vi "Vision Processing.vi"(4 "error in (no error)":errorcluster) -> ()   [LabVIEW 2011]
doc: "This VI runs in parallel to other tasks. It gets images from the camera, processes them for color or shape and use that information to affect robot behavior."
uses:
  <vilib>/vision/NI_Vision_Development_Module.lvlib
  VisionData.vi
  <vilib>/Rock Robotics/WPI/Camera/WPI_CameraImageSize.ctl
panel:
  in  "Color Mode":u16(ring)=1 items=["RGB", "HSL", "HSV", "HSI"]
  in  "Blue/Lum":cluster{"Lower value":i32, "Upper value":i32}={"Lower value"=40, "Upper value"=255}
  in  "Green/Sat":cluster{"Lower value":i32, "Upper value":i32}={"Lower value"=100, "Upper value"=255}
  in  "Red/hue":cluster{"Lower value":i32, "Upper value":i32}={"Lower value"=237, "Upper value"=8}
  in  "milliseconds to wait":u32=10
  out "x-y":u32
  in  "Compression":i32 min=0 max=100
  in  "Image Size":T1=enum."320x240"
  out "VisionClusterOut":T2
  out "Boolean":bool
  out "IRLLeft":bool
  out "IRLCenter":bool
  out "IRLRight":bool
  out "output array":bool[](array[boolean])
  out "error out":errorcluster
  in  "ActuallyDrawRectangles":bool
  in  "Enable/Disable Vision":bool=TRUE
  out "Scored Particle Info 3":T3(array[cluster])
  out "Scored Particle Info 2":T3(array[cluster])
  out "Scored Particle Info":T3(array[cluster])
  out "Processed Image 2":T4(plugin-control)
  in  "Score Limits":T5={"Rect Coverage"=60.0, "Aspect Ratio"=40.0, "X Edge Strength"=40.0, "Y Edge Strength"=60.0}
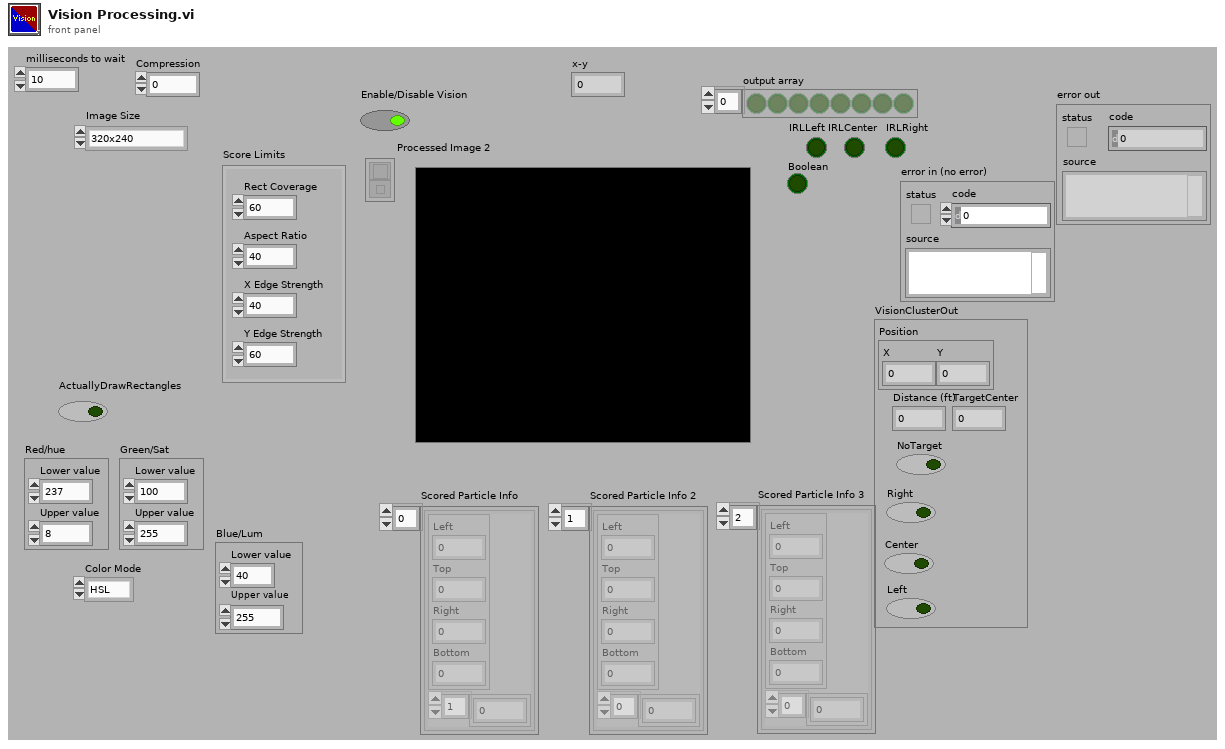
[diagram p1: front panel]
types:
  T1 = typedef "WPI_CameraImageSize.ctl" = enum16{"640x480", "320x240", "160x120"}
  T2 = cluster{"Position":cluster{"X":dbl, "Y":dbl}, "Distance (ft)":dbl, "NoTarget":bool, "Right":bool, "Center":bool, "Left":bool, "TargetCenter":dbl}
  T3 = cluster{cluster{"Left":dbl, "Top":dbl, "Right":dbl, "Bottom":dbl}, dbl[]}[]
  T4 = typedef "IMAQ Image.ctl" = refnum<image>
  T5 = cluster{"Rect Coverage":dbl, "Aspect Ratio":dbl, "X Edge Strength":dbl, "Y Edge Strength":dbl}
  T6 = typedef "Image Type" = u32
  T7 = typedef "WPI_CameraDevRef.ctl" = cluster{"Camera Address":string, "CameraStatus":errorcluster, "Acquire Image Notifier":refnum<notifier>}
  T8 = typedef "WPI_DigitalOutputDevRef.ctl" = cluster{"Digital Module":T9, "DIO Channel":T10, "DevStatus":errorcluster}
  T9 = typedef "FPGA_TypedefDigitalModule.ctl" = enum16{"Digital Module 1", "Digital Module 2"}
  T10 = typedef "FPGA_DIOChannel.ctl" = enum8{"DIO 1", "DIO 2", "DIO 3", "DIO 4", "DIO 5", "DIO 6", "DIO 7", "DIO 8", "DIO 9", "DIO 10", "DIO 11", "DIO 12", "DIO 13", "DIO 14", "Invalid"}
  T11 = cluster{"Position":cluster{"X":dbl, "Y":dbl}, "Distance (ft)":dbl, "NoTarget":bool, "Right":bool, "Center":bool, "Left":bool, "TargetCenter":dbl}[]
  T12 = cluster{"Avg. Horizontal ":dbl, "Avg Vertical":dbl}[]
  T13 = cluster{"Left":dbl, "Top":dbl, "Right":dbl, "Bottom":dbl}
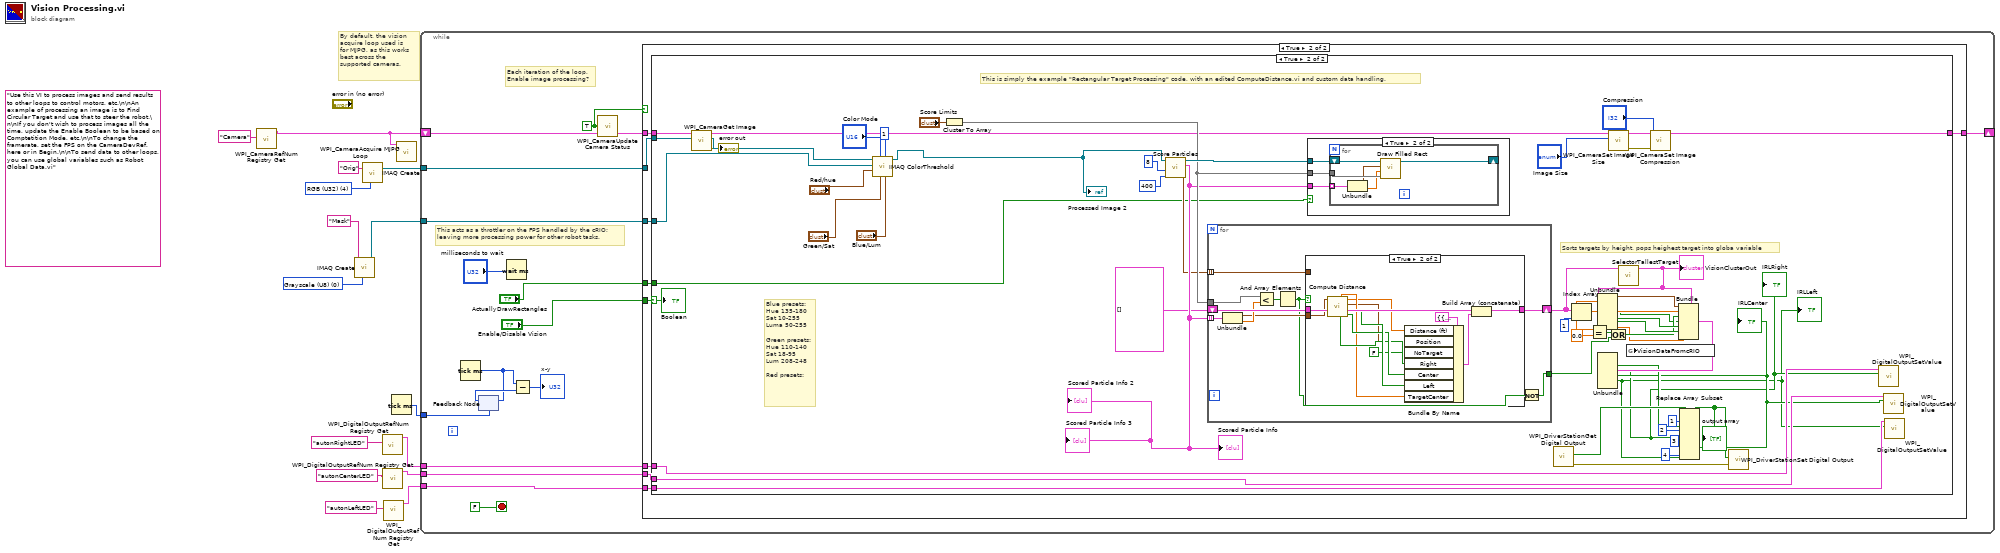
[diagram p0: block diagram]
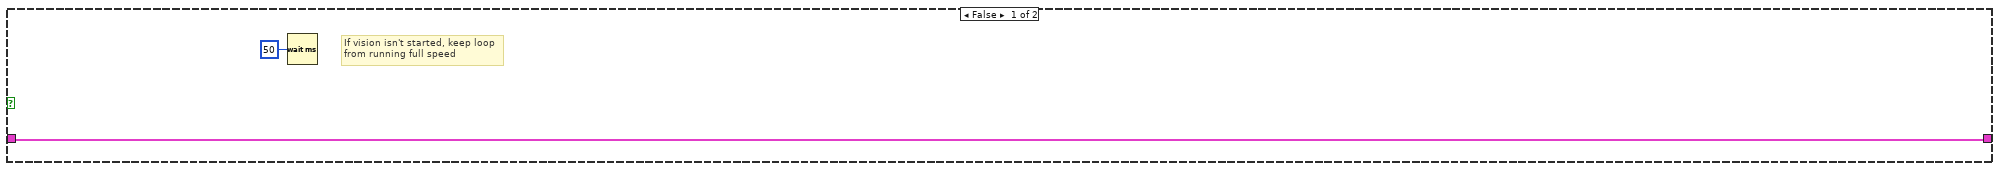
[diagram p2: hidden frame]
diagram:
  w11 = T6 0 items=["Grayscale (U8)", "Grayscale (I16)", "Grayscale (SGL)", "Complex (CSG)", "RGB (U32)", "HSL (U32)", "RGB (U64)"] ("Image Type")
  (unwired) "Use this VI to process images and send results to other loops to control motors, etc.\n\nAn example of processing an image is to Find Circular Target and use that to steer the robot.\n\nIf you don't wish to process images all the time, update the Enable Boolean to be based on Comptetition Mode, etc.\n\nTo change the framerate, set the FPS on the CameraDevRef, here or in Begin.\n\nTo send data to other loops, you can use global variables such as Robot Global Data.vi"
  w15 = T6 4 items=["Grayscale (U8)", "Grayscale (I16)", "Grayscale (SGL)", "Complex (CSG)", "RGB (U32)", "HSL (U32)", "RGB (U64)"] ("Image Type")
  # "By default, the vision\nacquire loop used is\nfor MJPG, as this works\nbest across the\nsupported cameras."
  n1 = call <vilib>:"WPI_CameraRefNum Registry Get.vi"("refnum name"="Camera") -> ("CameraDevRef"=w9:T7)  [unwired: 9 in, 1 out]
  n2 = call "IMAQ Create"("Image Name"="Mask", "Image Type"=w11) -> ("New Image"=w10:T4)  [unwired: 2 in, 2 out]
  n3 = call "IMAQ Create"("Image Name"="Orig", "Image Type"=w15) -> ("New Image"=w13:T4)  [unwired: 2 in, 2 out]
  n4 = call <vilib>:"WPI_DigitalOutputRefNum Registry Get.vi"("refnum name"="autonRightLED") -> ("DigitalOutputDevRef"=w4:T8)  [unwired: 9 in, 1 out]
  n5 = call <vilib>:"WPI_DigitalOutputRefNum Registry Get.vi"("refnum name"="autonCenterLED") -> ("DigitalOutputDevRef"=w3:T8)  [unwired: 9 in, 1 out]
  n6 = call <vilib>:"WPI_DigitalOutputRefNum Registry Get.vi"("refnum name"="autonLeftLED") -> ("DigitalOutputDevRef"=w2:T8)  [unwired: 9 in, 1 out]
  n7 = Tick Count (ms)() -> (millisecond timer value=w1:u32)
  n8 = call <vilib>:"WPI_CameraAcquire MJPG Loop.vi"("CameraDevRef"=w9) -> ()  [unwired: 11 in]
  n9 = while {
    shift-right: [w31] -> _
    shift-left: w9 -> [w29]
    tunnel: w13 -> [w30]
    tunnel: w10 -> [w28]
    tunnel: w4 -> [w24]
    tunnel: w3 -> [w23]
    tunnel: w2 -> [w22]
    tunnel: w1 -> [w20]
    stop <- FALSE stop-if-true
    w25 = TRUE ("Enable Vision")
    # "This acts as a throttler on the FPS handled by the cRIO;\nleaving more processing power for other robot tasks."
    # "Each iteration of the loop,\nEnable image processing?"
    n10 = Tick Count (ms)() -> (millisecond timer value=w18:u32)
    n11 = feedback-in #1(w18) -> ()
    n12 = feedback #1(w20) -> (w19:u32)
    n13 = Wait (ms)(milliseconds to wait="milliseconds to wait") -> ()  [unwired: 1 out]
    n14 = Subtract(x=w18, y=w19) -> (x-y=→"x-y":u32)
    n15 = call <vilib>:"WPI_CameraUpdate Camera Status.vi"("CameraDevRef In"=w29, "Enable Vision"=w25) -> ("CameraDevRef Out"=w27:T7)  [unwired: 3 in]
    n16 = case shown="True" w25 {
      tunnel: w30 -> [_ w42]
      tunnel: [w34 w43] -> w31
      tunnel: w27 -> [w34 w41]
      tunnel: w28 -> [_ w40]
      tunnel: "Enable/Disable Vision" -> [_ w39]
      tunnel: "ActuallyDrawRectangles" -> [_ w38]
      tunnel: w24 -> [_ w37]
      tunnel: w23 -> [_ w36]
      tunnel: w22 -> [_ w35]
      frame False {
        # "If vision isn't started, keep loop\nfrom running full speed"
        n17 = Wait (ms)(milliseconds to wait=u32 50) -> ()  [unwired: 1 out]
      }
      frame True {
        n18 = case shown="True" w39 {
          selector: w39 -> [_ w63]
          tunnel: [w44 w59] -> w43
          tunnel: w42 -> [_ w99]
          tunnel: w41 -> [w44 w98]
          tunnel: w40 -> [_ w97]
          tunnel: w38 -> [_ w88]
          tunnel: w37 -> [_ w71]
          tunnel: w36 -> [_ w73]
          tunnel: w35 -> [_ w72]
          frame False {
          }
          frame True {
            # "This is simply the example \"Rectangular Target Processing\" code, with an edited ComputeDistance.vi and custom data handling."
            # "Sorts targets by height, pops heighest target into globa variable"
            # "Blue presets:\nHue 135-180\nSat 10-255\nLuma 50-255\n\nGreen presets:\nHue 110-140\nSat 18-95\nLum 208-248\n\nRed presets:"
            n19 = call <vilib>:"WPI_CameraGet Image.vi"("Image"=w99, "CameraDevRef"=w98) -> ("error out"=→"error out":errorcluster, "Image Out"=w87:T4, "CameraDevRef Out"=w45:T7)  [unwired: 1 in, 6 out]
            n20 = call "IMAQ ColorThreshold"("Blue or Luma or Val or Inten Range"="Blue/Lum", "Replace Value"=1, "Green or Sat Range"="Green/Sat", "Color Mode"="Color Mode", "Red or Hue Range"="Red/hue", "Image Dst"=w97, "Image Src"=w87) -> ("Image Dst Out"=w53:T4)  [unwired: 3 in, 1 out]
            "Processed Image 2" <- w53
            n21 = Cluster To Array(cluster="Score Limits") -> (array=w92:dbl[])
            n22 = call "Score Particles.vi"("Area Size Limit"=400, "Particle Count Limit"=8, "Image Refnum in"=w53) -> ("Size Array"=w90:T12, "Scored Particle Info"=w91:T3, "Image Refnum out"=w93:T4)  [unwired: 6 in]
            "Scored Particle Info" <- w91
            "Scored Particle Info 2" <- w91
            "Scored Particle Info 3" <- w91
            n23 = for {
              shift-right: [w113] -> w55
              shift-left: T11 [] ("Array") -> [w118]
              tunnel: w92 -> [w115]
              tunnel: w91 -> [w114] mode=indexing
              tunnel: w90 -> [w109] mode=indexing
              tunnel: [w110] -> w67
              n24 = Unbundle(w114) -> (w112:T13, w116:dbl[])
              n25 = Less?(x=w115, y=w116) -> (x < y?=w117:bool[])
              n26 = And Array Elements(Boolean array=w117) -> (logical AND=w111:bool)
              n27 = case shown="True" w111 {
                tunnel: w118 -> [w119 w130]
                tunnel: [w119 w131] -> w113
                tunnel: w112 -> [_ w129]
                tunnel: w109 -> [_ _]
                frame False {
                }
                frame True {
                  n28 = call "Compute Distance.vi"("Bounding Box"=w129) -> ("Center"=w127:bool, "Right"=w128:bool, "Target Center (-1 to 1)"=w120:cluster{"X":dbl, "Y":dbl}, "Distance (ft)"=w121:dbl, "Left"=w126:bool, "-1 to 1 Center of Target Adjusted"=w124:dbl)  [unwired: 5 in]
                  n29 = Bundle By Name(cluster=T2 {"Position"={"X"=-1.0, "Y"=-1.0}, "Distance (ft)"=0.0, "NoTarget"=TRUE, "Right"=FALSE, "Center"=FALSE, "Left"=FALSE, "TargetCenter"=0.0} ("VisionData"), "Distance (ft)"=w121, "Position"=w120, "NoTarget"=FALSE, "Right"=w126, "Center"=w127, "Left"=w128, "TargetCenter"=w124) -> (w122:T2)
                  n30 = Build Array (concatenate)(w130, w122) -> (w131:T11)
                }
              }
              n31 = Not(x=w111) -> (.not. x?=w110:bool)
            }
            n32 = case shown="True" w88 {
              tunnel: w93 -> [_ w102]
              tunnel: w92 -> [_ w101]
              tunnel: w91 -> [_ w100]
              frame False {
              }
              frame True {
                n33 = for {
                  tunnel: w100 -> [w104] mode=indexing
                  tunnel: w101 -> [w108]
                  shift-right: [w106] -> _
                  shift-left: w102 -> [w105]
                  n34 = Unbundle(w104) -> (w107:T13, w103:dbl[])
                  n35 = call "Draw Filled Rect.vi"("Limits"=w108, "Scores"=w103, "Bounding Box"=w107, "image in"=w105) -> ("image out"=w106:T4)  [unwired: 7 in]
                }
              }
            }
            n36 = call <vilib>:"WPI_DriverStationGet Digital Output.vi"() -> ("error out"=w85:errorcluster, "Driver Station Digital Output (1-8)"=w84:bool[])  [unwired: 10 in]
            n37 = Index Array(array=w55, index=1) -> ()  [unwired: 1 out]
            n38 = call <vilib>:"WPI_CameraSet Image Size.vi"("Image Size"="Image Size", "CameraDevRef"=w45) -> ("error out"=w58:errorcluster, "CameraDevRef Out"=w60:T7)  [unwired: 1 in, 7 out]
            n39 = call "SelectorTallestTarget.vi"("Array"=w55) -> ("VisionClusterOut"=w74:T2)  [unwired: 9 in]
            "VisionClusterOut" <- w74
            n40 = Unbundle(w74) -> ("Position"=w78:cluster{"X":dbl, "Y":dbl}, "Distance (ft)"=w70:dbl, "Right"=w65:bool, "Center"=w76:bool, "Left"=w75:bool, "TargetCenter"=w62:dbl)  [unwired: 1 out]
            n41 = Equal?(x=w70, y=0.0) -> (x = y?=w68:bool)
            n42 = Or(x=w68, y=w67) -> (x .or. y?=w66:bool)
            n43 = call <vilib>:"WPI_CameraSet Image Compression.vi"("error in (no error)"=w58, "Compression"="Compression", "CameraDevRef"=w60) -> ("CameraDevRef Out"=w59:T7)  [unwired: 7 in, 1 out]
            n44 = Bundle(cluster=w74, "Position"=w78, "Distance (ft)"=w70, "NoTarget"=w66, "Right"=w65, "Center"=w76, "Left"=w75, "TargetCenter"=w62) -> (w77:T2)
            n45 = Unbundle(w77) -> ("NoTarget"=w64:bool, "Right"=w52:bool, "Center"=w56:bool, "Left"=w51:bool)  [unwired: 3 out]
            "IRLRight" <- w52
            "IRLCenter" <- w56
            "IRLLeft" <- w51
            n46 = global write "VisionData.vi" "VisionDataFromcRIO"(w77) -> ()
            n47 = Replace Array Subset(array=w84, new element #1=w64, index #1=1 ("index"), new element #2=w52, index #2=2 ("index"), new element #3=w56, index #3=3 ("index"), new element #4=w51, index #4=4 ("index")) -> (w83:bool[])
            "output array" <- w83
            n48 = call <vilib>:"WPI_DriverStationSet Digital Output.vi"("error in (no error)"=w85, "Driver Station Digital Output (1-8)"=w83) -> ()  [unwired: 9 in, 1 out]
            n49 = call <vilib>:"WPI_DigitalOutputSetValue.vi"("Value"=w52, "DigitalOutputDevRef"=w71) -> ()  [unwired: 8 in, 2 out]
            n50 = call <vilib>:"WPI_DigitalOutputSetValue.vi"("Value"=w56, "DigitalOutputDevRef"=w73) -> ()  [unwired: 8 in, 2 out]
            n51 = call <vilib>:"WPI_DigitalOutputSetValue.vi"("Value"=w51, "DigitalOutputDevRef"=w72) -> ()  [unwired: 8 in, 2 out]
            "Boolean" <- w63
          }
        }
      }
    }
  }
